vi "Post action.vi"(6 "Index":i32=41, 8 "error in (no error)":errorcluster, 9 "PostAction":T1=enum."Do Nothing", 10 "Scan Parameters":T2={"DAQ Channel"=3, "Label"="\nappliedVsg2=", "Start"=-0.01, "End"=0.4, "Step"=0.01, "Rate"=0.01, "VISA resource name"="", "wait (ms)"=10000} {"Rate" format="%.2f"; "Step" format="%#_6p"; "End" format="%#_6p"; "Start" format="%#_6p"}) -> (0 "error out":errorcluster)   [LabVIEW 2016, in "SweepControl.lvclass"]
uses:
  SweepControl.lvclass
  Typedefs/Cluster - ScanParamters.ctl
  Typedefs/Enum - PostAction.ctl
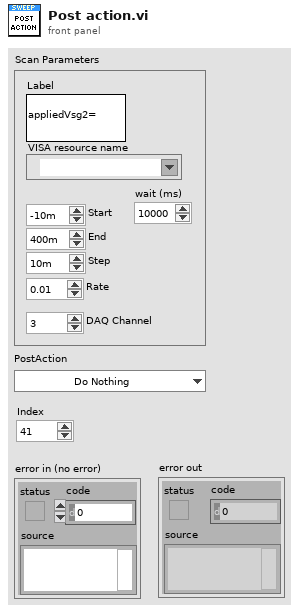
[diagram p1: front panel]
types:
  T1 = typedef "SweepControl.lvclass/Enum - PostAction.ctl" = enum16{"Clear DAQ Tasks", "Check Temperature", "Wait", "Do Nothing"}
  T2 = typedef "SweepControl.lvclass/Cluster - ScanParamters.ctl" = cluster{"DAQ Channel":i32, "Label":string, "Start":dbl, "End":dbl, "Step":dbl, "Rate":dbl, "VISA resource name":refnum<visa-resource-name>, "wait (ms)":u32}
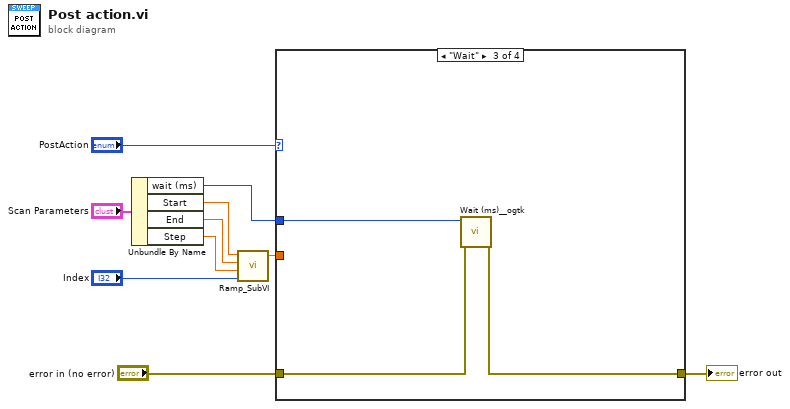
[diagram p0: block diagram]
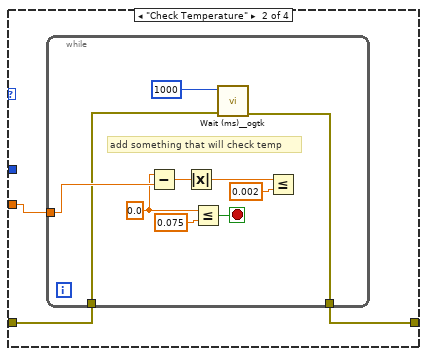
[diagram p3: hidden frame]
diagram:
  n1 = Unbundle By Name("Scan Parameters") -> ("wait (ms)"=w3:u32, "Start"=w6:dbl, "End"=w5:dbl, "Step"=w4:dbl)
  n2 = call <userlib>:"Ramp_SubVI.vi"("index"="Index", "step"=w4, "end"=w5, "start"=w6) -> ("Numeric"=w9:dbl)  [unwired: 1 in, 1 out]
  n3 = case shown="\"Wait\"" "PostAction" {
    tunnel: w9 -> [_ w14 _ _]
    tunnel: w3 -> [_ _ w27 _]
    tunnel: "error in (no error)" -> [w11 w13 w26 w28]
    tunnel: [w11 w12 w25 w28] -> w1
    frame .."Clear DAQ Tasks" {
      # "Not used anymore"
    }
    frame "Check Temperature" {
      n4 = while {
        tunnel: w14 -> [w21]
        tunnel: w13 -> [w16]
        tunnel: [w15] -> w12
        stop <- w19 stop-if-true
        w18 = 0.0 ("y")
        # "add something that will check temp"
        n5 = Subtract(x=w18, y=w21) -> (x-y=w24:dbl)
        n6 = Absolute Value(x=w24) -> (abs(x)=w23:dbl)
        n7 = Less Or Equal?(x=w18, y=0.075) -> (x <= y?=w19:bool)
        n8 = call <userlib>:"Wait (ms)__ogtk.vi"("error in (no error)"=w16, "milliseconds to wait"=u32 1000) -> ("error out"=w15:errorcluster)  [unwired: 8 in, 1 out]
        n9 = Less Or Equal?(x=w23, y=0.002) -> ()  [unwired: 1 out]
      }
    }
    frame "Wait" {
      n10 = call <userlib>:"Wait (ms)__ogtk.vi"("error in (no error)"=w26, "milliseconds to wait"=w27) -> ("error out"=w25:errorcluster)  [unwired: 8 in, 1 out]
    }
    frame "Do Nothing".. {
      # "Do nothing"
    }
  }
  "error out" <- w1
